vi "delay_5_minutes.vi"(8 "error in (no error)":errorcluster, 10 "start point":dbl, 11 ".NET Refnum in":refnum<k24>) -> (0 "error out":errorcluster, 3 ".NET Refnum out":refnum<k24>)   [LabVIEW 2015]
uses:
  C:/Program Files/National Instruments/LabVIEW 2015/vi.lib/ULx/ULx_LV.dll
  <vilib>/ULx/Write.llb/ULx Write (Analog 1D DBL 1Chan 1Samp).vi
  global_stop_calibration.vi
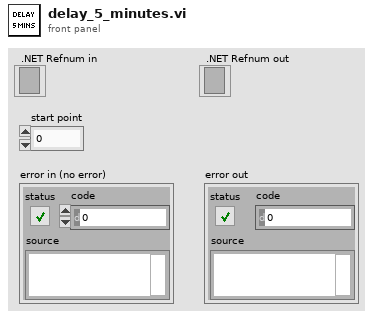
[diagram p1: front panel]
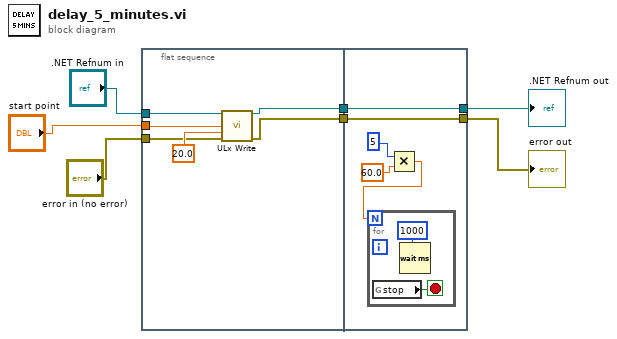
[diagram p0: block diagram]
diagram:
  n1 = flat-sequence {
    tunnel: [w12] -> w7
    tunnel: ".NET Refnum in" -> [w11]
    tunnel: "error in (no error)" -> [w10]
    tunnel: [w9] -> w6
    tunnel: "start point" -> [w8]
    tunnel: [w18] -> w2
    tunnel: w7 -> [w18]
    tunnel: w6 -> [w17]
    tunnel: [w17] -> w3
    frame #0 {
      n2 = call-poly <vilib>:"ULx Write.vi"("task in"=w11, "data"=w8, "timeout"=20.0, "error in"=w10) -> ("task out"=w12:refnum<k24>, "error out"=w9:errorcluster)  [unwired: 9 in, 1 out]
    }
    frame #1 {
      n3 = Multiply(x=5, y=60.0) -> (x*y=w14:dbl)
      n4 = for {
        N: w14 -> [_]
        stop <- w20 stop-if-true
        n5 = global read "global_stop_calibration.vi" "stop"() -> (w20:bool)
        n6 = Wait (ms)(milliseconds to wait=u32 1000) -> ()  [unwired: 1 out]
      }
    }
  }
  ".NET Refnum out" <- w2
  "error out" <- w3
